vi "Reverse 1D Array.vi"(8 "error in (no error)":errorcluster, 11 "JSON Value in":refnum<class "JSON Value.lvclass">) -> (0 "error out":errorcluster, 3 "JSON Value out":refnum<class "JSON Value.lvclass">)   [LabVIEW 2016, in "JSON Value.lvclass"]
doc: "Reverses the order of the elements in array, where array is of any type."
uses:
  JSON Value.lvclass
  JSON Value.lvclass/JSON Value.ctl
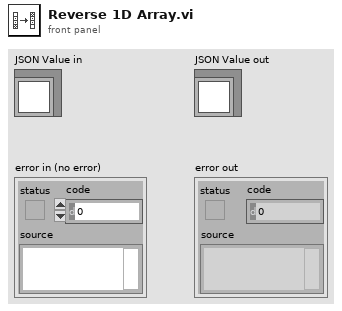
[diagram p1: front panel]
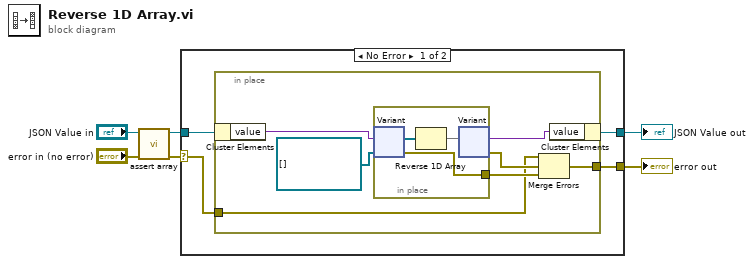
[diagram p0: block diagram]
diagram:
  n1 = call "assert array.vi"("error in (no error)"="error in (no error)", "JSON Value in"="JSON Value in") -> ("error out"=w2:errorcluster, "JSON Value out"=w4:refnum<class "JSON Value.lvclass">)  [unwired: 8 in]
  n2 = case shown="No Error" w2 {
    selector: w2 -> [w7 w21]
    tunnel: [w10 w22] -> w5
    tunnel: w4 -> [w9 w22]
    tunnel: [w8 w21] -> w1
    frame No Error {
      n3 = in-place {
        in-place-border: [w12] -> w8
        in-place-border: w7 -> [w11]
        n4 = in-place-cluster #1(w9) -> ("value"=w16:variant)
        n5 = in-place {
          in-place-border: [w18] -> w13
          n6 = in-place-variant #2(w16, refnum<class "JSON Value.lvclass">[] [] ("JSON Value in")) -> (w20:refnum<class "JSON Value.lvclass">[], w18:errorcluster)
          n7 = Reverse 1D Array(array=w20) -> (reversed array=w19:refnum<class "JSON Value.lvclass">[])
          n8 = in-place-variant #2(w19) -> (w15:variant, w14:errorcluster)
        }
        n9 = Merge Errors(w11, w14, w13) -> (w12:errorcluster)
        n10 = in-place-cluster #1("value"=w15) -> (w10:refnum<class "JSON Value.lvclass">)
      }
    }
    frame Error {
    }
  }
  "JSON Value out" <- w5
  "error out" <- w1
